vi "0805_Controle_FMS.vi"() -> ()   [LabVIEW 2017]
uses:
  <vilib>/myRIO/Instrument Drivers/Onboard IO/PWM/typedefs/PWM Reference.ctl
  <vilib>/myRIO/Common/Instrument Driver Framework/Utilities/typedefs/myRIO Generic Hardware Reference.ctl
  <vilib>/myRIO/Common/Instrument Driver Framework/Utilities/typedefs/Hardware Version Enum.ctl
  <vilib>/myRIO/Common/Instrument Driver Framework/Utilities/typedefs/myRIO v1.0 Reference.ctl
  <vilib>/myRIO/Common/Instrument Driver Framework/Utilities/typedefs/Generic FPGA Reference.ctl
  <vilib>/myRIO/Common/Instrument Driver Framework/myRIO v1.0/PWM/typedefs/PWM Channels Enum.ctl
  <vilib>/myRIO/Instrument Drivers/Onboard IO/PWM/typedefs/PWM Configuration.ctl
  <vilib>/userdefined/High Color/nirio_resource_hc.ctl
  <vilib>/myRIO/Common/Instrument Driver Framework/myRIO v1.0/PWM/vis/myRIO v1.1 Open PWM.vi
  <vilib>/myRIO/Common/Instrument Driver Framework/Utilities/vis/Validate Channels.vi
  <vilib>/myRIO/Common/Instrument Driver Framework/myRIO v1.0/PWM/vis/myRIO v1.0 Reserve PWM.vi
  <vilib>/myRIO/Instrument Drivers/Onboard IO/PWM/vis/Set Duty Cycle and Frequency.vi
  <vilib>/myRIO/Common/Instrument Driver Framework/myRIO v1.0/PWM/vis/myRIO v1.0 Close PWM.vi
  <vilib>/myRIO/Common/Instrument Driver Framework/myRIO v1.0/PWM/vis/myRIO v1.0 Build MUX Configuration PWM.vi
  <vilib>/myRIO/Common/Instrument Driver Framework/myRIO v1.0/Resource Manager/vis/myRIO v1.0 Reserve Channel List.vi
  <vilib>/myRIO/Common/Instrument Driver Framework/myRIO v1.0/PWM/vis/myRIO v1.0 Unreserve PWM.vi
  <vilib>/myRIO/Common/Instrument Driver Framework/myRIO v1.0/Resource Manager/vis/myRIO v1.0 Create Configuration List.vi
  <vilib>/myRIO/Common/Instrument Driver Framework/myRIO v1.0/Resource Manager/vis/myRIO v1.0 Reserve Channel.vi
  <vilib>/myRIO/Common/Instrument Driver Framework/myRIO v1.0/Resource Manager/vis/myRIO v1.0 Unreserve Channel.vi
  <vilib>/myRIO/Common/Instrument Driver Framework/myRIO v1.0/Resource Manager/vis/myRIO v1.0 Unreserve Channel List.vi
  <vilib>/myRIO/Common/Instrument Driver Framework/myRIO v1.0/Resource Manager/vis/myRIO v1.0 Build Mutex Name.vi
  <vilib>/Utility/VariantDataType/GetNumericInfo.vi
  <vilib>/Utility/error.llb/Error Cluster From Error Code.vi
  <vilib>/myRIO/Common/Instrument Driver Framework/myRIO v1.0/myRIO v1.1 Open.vi
  <vilib>/myRIO/Common/Instrument Driver Framework/Utilities/vis/IO Manager.vi
  <vilib>/myRIO/Common/Instrument Driver Framework/Utilities/vis/Configuration Manager.vi
  <vilib>/myRIO/Common/Instrument Driver Framework/myRIO v1.0/Resource Manager/vis/myRIO v1.0 Configure IO.vi
  <vilib>/myRIO/Common/Instrument Driver Framework/myRIO v1.0/myRIO v1.0 Close.vi
  <vilib>/myRIO/Common/Instrument Driver Framework/myRIO v1.0/PWM/vis/myRIO v1.0 Write PWM.vi
  <vilib>/myRIO/Common/Instrument Driver Framework/myRIO v1.0/PWM/vis/myRIO v1.0 Shutdown PWM.vi
  <vilib>/myRIO/Instrument Drivers/Onboard IO/PWM/vis/myRIO PWM Open.xnode
  <vilib>/myRIO/Instrument Drivers/Onboard IO/PWM/PWM.lvlib
panel:
  out "Parar_esteira":bool
  out "Objeto_detectado":bool
  out "Actuator 2":bool
  in  "delay between positions (ms)":u32=5
  out "Manipulating":bool
  out "Ready_to_manipulate":bool
  out "Is_position_desired":bool
  out "Is_robot_home":bool
  out "Local_stop":bool
  out "ms":u32
  in  "Stop conveyor":bool=TRUE
  in  "Conveyor speed (mm/s)":dbl(slide)=200.0 step=1.0 scale=0.0..350.0
  in  "Actuator":bool
  in  "Positions_control":u16(ring) items=["Livre", "Posição 1", "Posição 2", "Posição 3", "Posição 4", "Posição 5", "Posição 6", "Posição 7", "Fim"]
  in  "Stop":bool
  out "Position":dbl[](array[knob]) scale=0.0..200.0
  in  "Desired position":dbl[](array[slide])=[0.0, -180.0, 30.0, -60.0, -60.0, -60.0] min=-180.0 max=180.0 step=1.0 scale=-270.0..270.0
  in  "Home":bool
  out "error out":errorcluster
  in  "error in (no error)":errorcluster
  in  "ms to wait (braço)":u32=5
  # "Range: 0,025 - 0,125\n\n3° = 0,00125\n\nLink 1 - (0,00125/3)x + 0,1\n0,125 -> 60°\n0,1 -> 0°\n0,0625 -> -90\n0,025 -> -180°\n\nLink 2 - -(0,00125/3)x + 0,1\n0,025 -> 180°\n0,0625 -> 90°\n0,1 -> 0°\n0,125 -> -60°\n\nLink 3 - (0,00125/3)x - 0,0125\n0,125 -> 300°\n0,105 -> 270° \n0,63 -> 180°\n0,025 -> 90°\n\n9° = 0,05\n\nLink 5 - (0,005/9)x + 0,075\n0,125 -> 90°\n0,075 -> 0°\n0,025 ->-90°"
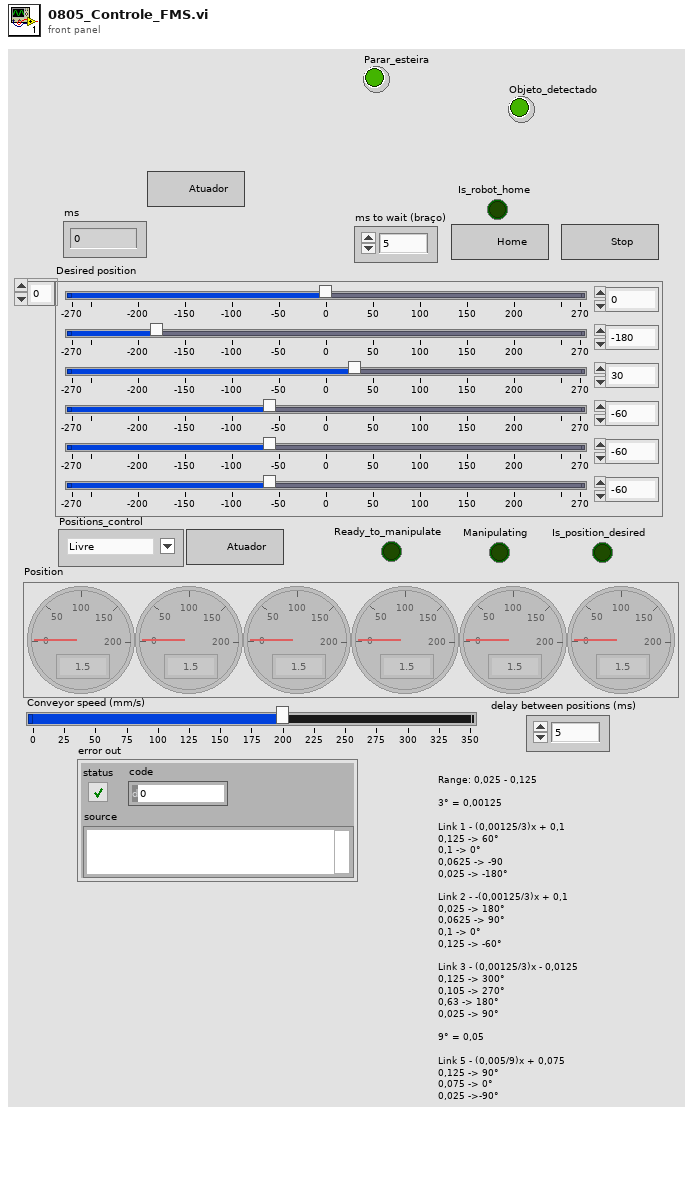
[diagram p1: front panel]
types:
  T1 = typedef "nirio_resource_hc.ctl" = tag
  T2 = typedef "Hardware Version Enum.ctl" = enum16{"Unknown", "myRIO-1900", "myRIO-1950", "roboRIO", "NI ELVIS RIO CM"}
  T3 = typedef "PWM.lvlib/PWM Reference.ctl" = cluster{"myRIO Reference":T4, "PWM Channels Enum":T7, "PWM Configuration":T8}
  T4 = typedef "myRIO Generic Hardware Reference.ctl" = cluster{"myRIO Model":T2, "myRIO Hardware Reference":T5}
  T5 = typedef "myRIO v1.0 Reference.ctl" = cluster{"Generic FPGA Reference":T6, "Allow multiple opens":bool}
  T6 = typedef "Generic FPGA Reference.ctl" = refnum<k20>
  T7 = typedef "PWM Channels Enum.ctl" = enum16{"Not Connected", "C/PWM0", "C/PWM1", "A/PWM0", "A/PWM1", "A/PWM2", "B/PWM0", "B/PWM1", "B/PWM2", "PWM/PWM0", "PWM/PWM1", "PWM/PWM2", "PWM/PWM3", "PWM/PWM4", "PWM/PWM5", "PWM/PWM6", "PWM/PWM7", "PWM/PWM8", "PWM/PWM9"}
  T8 = typedef "PWM.lvlib/PWM Configuration.ctl" = cluster{"Frequency":dbl, "Duty Cycle":dbl}
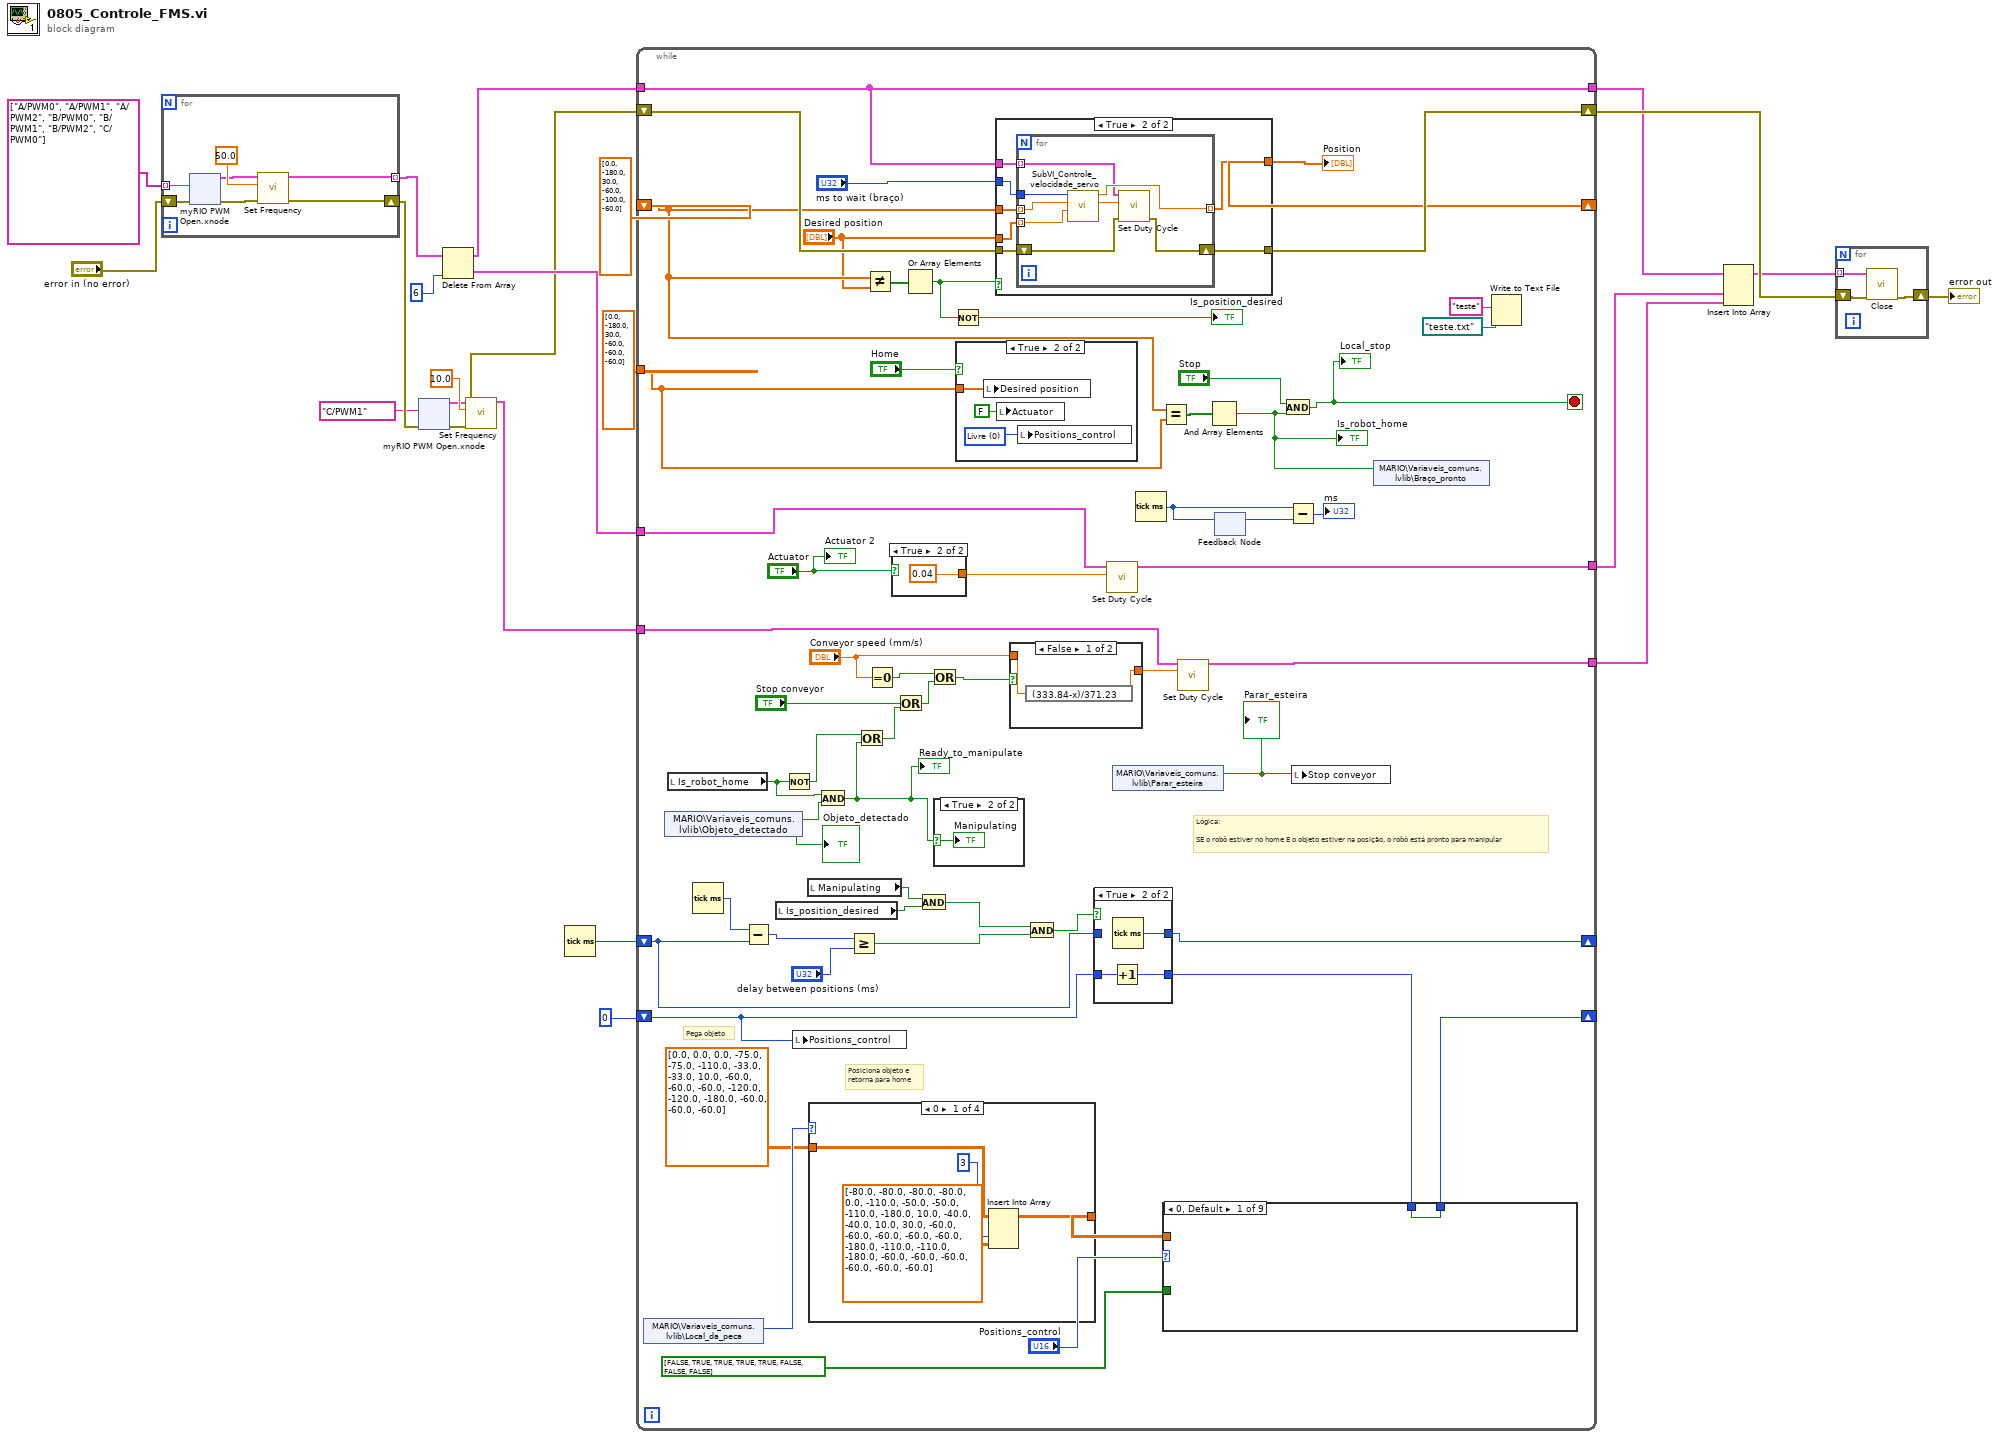
[diagram p0: block diagram]
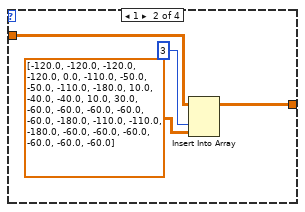
[diagram p2: hidden frame]
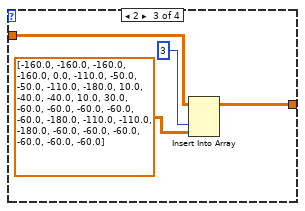
[diagram p3: hidden frame]
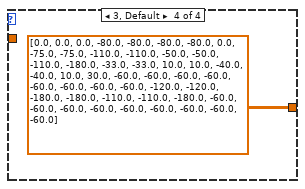
[diagram p4: hidden frame]
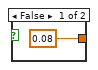
[diagram p8: hidden frame]
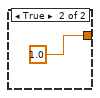
[diagram p10: hidden frame]
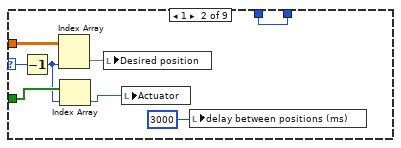
[diagram p11: hidden frame]
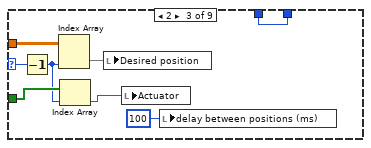
[diagram p12: hidden frame]
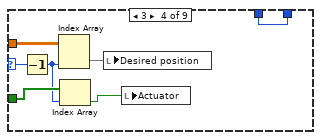
[diagram p13: hidden frame]
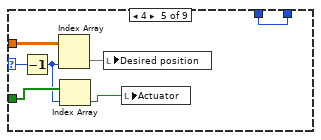
[diagram p14: hidden frame]
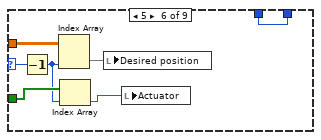
[diagram p15: hidden frame]
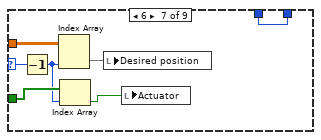
[diagram p16: hidden frame]
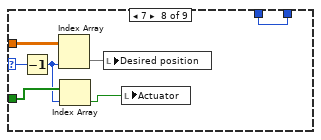
[diagram p17: hidden frame]
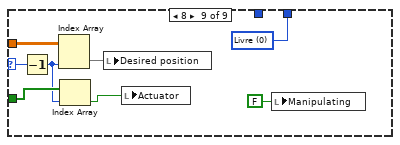
[diagram p18: hidden frame]
diagram:
  n1 = for {
    shift-right: [w24] -> w13
    shift-left: "error in (no error)" -> [w29]
    tunnel: tag[] ["A/PWM0", "A/PWM1", "A/PWM2", "B/PWM0", "B/PWM1", "B/PWM2", "C/PWM0"] -> [w30] mode=indexing
    tunnel: [w25] -> w10 mode=indexing
    n2 = xnode ("myRIO PWM Open.xnode")("error in (no error)"=w29, "Channel Name"=w30) -> ("error out"=w27:errorcluster, "PWM Ref Out"=w26:T3)  [unwired: 1 in]
    n3 = call <vilib>:"Set Frequency.vi"("error in (no error)"=w27, "Frequency [Hz]"=50.0, "PWM Ref In"=w26) -> ("error out"=w24:errorcluster, "PWM Ref Out"=w25:T3)  [unwired: 6 in]
  }
  n4 = xnode "myRIO PWM Open.xnode"("error in (no error)"=w13, "Channel Name"=tag "C/PWM1") -> ("error out"=w14:errorcluster, "PWM Ref Out"=w15:T3)  [unwired: 1 in]
  n5 = Delete From Array(array=w10, index=6) -> (deleted portion=w7:T3, array with subset deleted=w8:T3[])  [unwired: 1 in]
  n6 = call <vilib>:"Set Frequency.vi"("error in (no error)"=w14, "Frequency [Hz]"=10.0, "PWM Ref In"=w15) -> ("error out"=w6:errorcluster, "PWM Ref Out"=w5:T3)  [unwired: 6 in]
  n7 = Tick Count (ms)() -> (millisecond timer value=w2:u32)
  n8 = while {
    shift-right: [w101] -> w23
    shift-left: w6 -> [w102]
    shift-right: [w100] -> _
    shift-left: dbl[] [0.0, -180.0, 30.0, -60.0, -100.0, -60.0] -> [w82]
    tunnel: w8 -> [w99]
    tunnel: [w99] -> w20
    tunnel: dbl[] [0.0, -180.0, 30.0, -60.0, -60.0, -60.0] -> [w95]
    tunnel: w7 -> [w93]
    tunnel: [w91] -> w19
    tunnel: w5 -> [w89]
    tunnel: [w87] -> w17
    shift-right: [w61] -> _
    shift-left: w2 -> [w62]
    shift-right: [w58] -> _
    shift-left: 0 -> [w60]
    stop <- w79 stop-if-true
    # "Lógica:\n\nSE o robô estiver no home E o objeto estiver na posição, o robô está pronto para manipular"
    # "Posiciona objeto e \nretorna para home"
    # "Pega objeto"
    n9 = shared-variable "MARIO\\Variaveis_comuns.lvlib\\Local_da_peca"() -> (w53:i8)  [unwired: 1 in, 1 out]
    n10 = shared-variable "MARIO\\Variaveis_comuns.lvlib\\Objeto_detectado"() -> (w75:bool)  [unwired: 1 in, 1 out]
    "Objeto_detectado" <- w75
    n11 = local read "Is_robot_home"() -> (w74:bool)
    n12 = Tick Count (ms)() -> (millisecond timer value=w66:u32)
    n13 = Subtract(x=w66, y=w62) -> (x-y=w65:u32)
    n14 = local read "Is_position_desired"() -> (w56:bool)
    n15 = Not(x=w74) -> (.not. x?=w73:bool)
    n16 = local write "Positions_control"(w60) -> ()
    n17 = local read "Manipulating"() -> (w57:bool)
    n18 = case shown="0" w53 {
      tunnel: dbl[][] [[0.0, 0.0, 0.0], [-75.0, -75.0, -110.0], [-33.0, -33.0, 10.0], [-60.0, -60.0, -60.0], [-120.0, -120.0, -180.0], [-60.0, -60.0, -60.0]] ("Positions") -> [w105 w111 w115 _]
      tunnel: [w104 w110 w113 dbl[][] [[0.0, 0.0, 0.0, -80.0, -80.0, -80.0, -80.0, 0.0], [-75.0, -75.0, -110.0, -110.0, -50.0, -50.0, -110.0, -180.0], [-33.0, -33.0, 10.0, 10.0, -40.0, -40.0, 10.0, 30.0], [-60.0, -60.0, -60.0, -60.0, -60.0, -60.0, -60.0, -60.0], [-120.0, -120.0, -180.0, -180.0, -110.0, -110.0, -180.0, -60.0], [-60.0, -60.0, -60.0, -60.0, -60.0, -60.0, -60.0, -60.0]] ("Positions")] -> w49
      frame 0 {
        n19 = Insert Into Array(array=w105, index (col)=3 ("disabled index (col)"), new element=dbl[][] [[-80.0, -80.0, -80.0, -80.0, 0.0], [-110.0, -50.0, -50.0, -110.0, -180.0], [10.0, -40.0, -40.0, 10.0, 30.0], [-60.0, -60.0, -60.0, -60.0, -60.0], [-180.0, -110.0, -110.0, -180.0, -60.0], [-60.0, -60.0, -60.0, -60.0, -60.0]] ("Positions")) -> (w104:dbl[][])  [unwired: 1 in]
      }
      frame 1 {
        n20 = Insert Into Array(array=w111, index (col)=3 ("disabled index (col)"), new element=dbl[][] [[-120.0, -120.0, -120.0, -120.0, 0.0], [-110.0, -50.0, -50.0, -110.0, -180.0], [10.0, -40.0, -40.0, 10.0, 30.0], [-60.0, -60.0, -60.0, -60.0, -60.0], [-180.0, -110.0, -110.0, -180.0, -60.0], [-60.0, -60.0, -60.0, -60.0, -60.0]] ("Positions")) -> (w110:dbl[][])  [unwired: 1 in]
      }
      frame 2 {
        n21 = Insert Into Array(array=w115, index (col)=3 ("disabled index (col)"), new element=dbl[][] [[-160.0, -160.0, -160.0, -160.0, 0.0], [-110.0, -50.0, -50.0, -110.0, -180.0], [10.0, -40.0, -40.0, 10.0, 30.0], [-60.0, -60.0, -60.0, -60.0, -60.0], [-180.0, -110.0, -110.0, -180.0, -60.0], [-60.0, -60.0, -60.0, -60.0, -60.0]] ("Positions")) -> (w113:dbl[][])  [unwired: 1 in]
      }
      frame 3, Default {
      }
    }
    n22 = And(x=w74, y=w75) -> (x .and. y?=w68:bool)
    "Ready_to_manipulate" <- w68
    n23 = Greater Or Equal?(x=w65, y="delay between positions (ms)") -> (x >= y?=w64:bool)
    n24 = Or(x=w73, y=w68) -> (x .or. y?=w72:bool)
    n25 = Not Equal?(x=w82, y="Desired position") -> (x != y?=w80:bool[])
    n26 = Equal To 0?(x="Conveyor speed (mm/s)") -> (x = 0?=w78:bool)
    n27 = case shown="True" "Actuator" {
      tunnel: [0.08 ("Duty Cycle Abert") 0.04 ("Duty Cycle Abert")] -> w92
      frame False {
      }
      frame True {
      }
    }
    n28 = Or(x="Stop conveyor", y=w72) -> (x .or. y?=w76:bool)
    n29 = Or Array Elements(Boolean array=w80) -> (logical OR=w71:bool)
    n30 = And(x=w57, y=w56) -> (x .and. y?=w55:bool)
    n31 = Or(x=w78, y=w76) -> (x .or. y?=w86:bool)
    n32 = case shown="True" w68 {
      selector: w68 -> [_ w122]
      frame False {
      }
      frame True {
        "Manipulating" <- w122
      }
    }
    n33 = Not(x=w71) -> (.not. x?=→"Is_position_desired":bool)
    n34 = case shown="True" "Home" {
      tunnel: w95 -> [_ w144]
      frame False {
      }
      frame True {
        w142 = u16 0 items=["Livre", "Posição 1", "Posição 2", "Posição 3", "Posição 4", "Posição 5"] ("Menu Ring")
        n35 = local write "Desired position"(w144) -> ()
        n36 = local write "Actuator"(FALSE ("Atuador")) -> ()
        n37 = local write "Positions_control"(w142) -> ()
      }
    }
    n38 = case shown="True" w71 {
      tunnel: "ms to wait (braço)" -> [_ w131]
      tunnel: "Desired position" -> [_ w130]
      tunnel: w102 -> [w124 w129]
      tunnel: [w124 w128] -> w101
      tunnel: [w123 w127] -> w100
      tunnel: w99 -> [_ w126]
      tunnel: w82 -> [w123 w125]
      frame False {
      }
      frame True {
        n39 = for {
          tunnel: w131 -> [w139]
          tunnel: w126 -> [w134] mode=indexing
          tunnel: w130 -> [w132] mode=indexing
          tunnel: w125 -> [w133] mode=indexing
          shift-right: [w135] -> w128
          shift-left: w129 -> [w136]
          tunnel: [w138] -> w127 mode=indexing
          n40 = call "SubVI_Controle_velocidade_servo.vi"("Posição Desejada"=w132, "Posição"=w133, "milliseconds to wait"=w139) -> ("Duty Cycle"=w137:dbl, "Posição"=w138:dbl)  [unwired: 7 in]
          n41 = call <vilib>:"Set Duty Cycle.vi"("error in (no error)"=w136, "Duty Cycle"=w137, "PWM Ref In"=w134) -> ("error out"=w135:errorcluster)  [unwired: 6 in, 1 out]
        }
      }
    }
    "Position" <- w100
    n42 = case shown="False" w86 {
      tunnel: [w145 1.0] -> w88
      tunnel: "Conveyor speed (mm/s)" -> [w146 _]
      frame False {
        n43 = expression code="(333.84-x)/371.23"(w146) -> (w145:dbl)
      }
      frame True {
      }
    }
    n44 = And(x=w55, y=w64) -> (x .and. y?=w63:bool)
    n45 = case shown="True" w63 {
      tunnel: w62 -> [w118 _]
      tunnel: [w118 w121] -> w61
      tunnel: w60 -> [w117 w120]
      tunnel: [w117 w119] -> w59
      frame False {
      }
      frame True {
        n46 = Increment(x=w120) -> (x+1=w119:i32)
        n47 = Tick Count (ms)() -> (millisecond timer value=w121:u32)
      }
    }
    n48 = call <vilib>:"Set Duty Cycle.vi"("Duty Cycle"=w92, "PWM Ref In"=w93) -> ("PWM Ref Out"=w91:T3)  [unwired: 7 in, 1 out]
    n49 = shared-variable "MARIO\\Variaveis_comuns.lvlib\\Parar_esteira"() -> (w52:bool)  [unwired: 1 in, 1 out]
    "Parar_esteira" <- w52
    n50 = Tick Count (ms)() -> (millisecond timer value=w84:u32)
    n51 = Equal?(x=w82, y=w95) -> (x = y?=w96:bool[])
    n52 = case shown="0, Default" "Positions_control" {
      selector: "Positions_control" -> [_ w154 w162 w169 w176 w183 w190 w197 w205]
      tunnel: w49 -> [_ w156 w164 w171 w178 w185 w192 w199 w207]
      tunnel: bool[] [FALSE, TRUE, TRUE, TRUE, TRUE, FALSE, FALSE, FALSE] ("Actuator_positions") -> [_ w153 w161 w168 w175 w182 w189 w196 w204]
      tunnel: w59 -> [w148 w150 w158 w165 w172 w179 w186 w193 _]
      tunnel: [w148 w150 w158 w165 w172 w179 w186 w193 w200] -> w58
      frame 0, Default {
      }
      frame 1 {
        n53 = Decrement(x=w154) -> (x-1=w152:u16)
        n54 = Index Array(array=w156, index (col)=w152) -> (element=w155:dbl[])  [unwired: 1 in]
        n55 = Index Array(array=w153, index=w152) -> (element=w151:bool)
        n56 = local write "Desired position"(w155) -> ()
        n57 = local write "Actuator"(w151) -> ()
        n58 = local write "delay between positions (ms)"(u32 3000 ("delay between positions (ms)")) -> ()
      }
      frame 2 {
        n59 = Decrement(x=w162) -> (x-1=w160:u16)
        n60 = Index Array(array=w164, index (col)=w160) -> (element=w163:dbl[])  [unwired: 1 in]
        n61 = Index Array(array=w161, index=w160) -> (element=w159:bool)
        n62 = local write "Desired position"(w163) -> ()
        n63 = local write "Actuator"(w159) -> ()
        n64 = local write "delay between positions (ms)"(u32 100 ("delay between positions (ms)")) -> ()
      }
      frame 3 {
        n65 = Decrement(x=w169) -> (x-1=w167:u16)
        n66 = Index Array(array=w171, index (col)=w167) -> (element=w170:dbl[])  [unwired: 1 in]
        n67 = Index Array(array=w168, index=w167) -> (element=w166:bool)
        n68 = local write "Desired position"(w170) -> ()
        n69 = local write "Actuator"(w166) -> ()
      }
      frame 4 {
        n70 = Decrement(x=w176) -> (x-1=w174:u16)
        n71 = Index Array(array=w178, index (col)=w174) -> (element=w177:dbl[])  [unwired: 1 in]
        n72 = Index Array(array=w175, index=w174) -> (element=w173:bool)
        n73 = local write "Desired position"(w177) -> ()
        n74 = local write "Actuator"(w173) -> ()
      }
      frame 5 {
        n75 = Decrement(x=w183) -> (x-1=w181:u16)
        n76 = Index Array(array=w185, index (col)=w181) -> (element=w184:dbl[])  [unwired: 1 in]
        n77 = Index Array(array=w182, index=w181) -> (element=w180:bool)
        n78 = local write "Desired position"(w184) -> ()
        n79 = local write "Actuator"(w180) -> ()
      }
      frame 6 {
        n80 = Decrement(x=w190) -> (x-1=w188:u16)
        n81 = Index Array(array=w192, index (col)=w188) -> (element=w191:dbl[])  [unwired: 1 in]
        n82 = Index Array(array=w189, index=w188) -> (element=w187:bool)
        n83 = local write "Desired position"(w191) -> ()
        n84 = local write "Actuator"(w187) -> ()
      }
      frame 7 {
        n85 = Decrement(x=w197) -> (x-1=w195:u16)
        n86 = Index Array(array=w199, index (col)=w195) -> (element=w198:dbl[])  [unwired: 1 in]
        n87 = Index Array(array=w196, index=w195) -> (element=w194:bool)
        n88 = local write "Desired position"(w198) -> ()
        n89 = local write "Actuator"(w194) -> ()
      }
      frame 8 {
        w200 = u16 0 items=["Livre", "Posição 1", "Posição 2", "Posição 3", "Posição 4", "Posição 5", "Posição 6", "Posição 7", "Fim"] ("Positions_control")
        n90 = Decrement(x=w205) -> (x-1=w203:u16)
        n91 = Index Array(array=w207, index (col)=w203) -> (element=w206:dbl[])  [unwired: 1 in]
        n92 = Index Array(array=w204, index=w203) -> (element=w202:bool)
        n93 = local write "Desired position"(w206) -> ()
        n94 = local write "Actuator"(w202) -> ()
        n95 = local write "Manipulating"(FALSE ("Manipulating")) -> ()
      }
    }
    n96 = call <vilib>:"Set Duty Cycle.vi"("Duty Cycle"=w88, "PWM Ref In"=w89) -> ("PWM Ref Out"=w87:T3)  [unwired: 7 in, 1 out]
    n97 = And Array Elements(Boolean array=w96) -> (logical AND=w51:bool)
    "Is_robot_home" <- w51
    n98 = feedback-in #1(w84) -> ()
    n99 = feedback #1() -> (w83:u32)  [unwired: 1 in]
    n100 = And(x="Stop", y=w51) -> (x .and. y?=w79:bool)
    "Local_stop" <- w79
    n101 = Subtract(x=w84, y=w83) -> (x-y=→"ms":u32)
    n102 = local write "Stop conveyor"(w52) -> ()
    n103 = shared-variable "MARIO\\Variaveis_comuns.lvlib\\Braço_pronto"(w51) -> ()  [unwired: 1 in, 1 out]
    n104 = Write to Text File(file (use dialog)=path "/teste.txt", text="teste") -> ()  [unwired: 2 in, 3 out]
    "Actuator 2" <- "Actuator"
  }
  n105 = Insert Into Array(array=w20, new element #1=w19, new element #2=w17) -> (w18:T3[])  [unwired: 1 in]
  n106 = for {
    tunnel: w18 -> [w210] mode=indexing
    shift-right: [w208] -> w22
    shift-left: w23 -> [w209]
    n107 = call <vilib>:"Close.vi"("error in (no error)"=w209, "PWM Ref In"=w210) -> ("error out"=w208:errorcluster)  [unwired: 9 in]
  }
  "error out" <- w22
